vi "Write Options.vi"(8 "error in (no error)":errorcluster, 10 "WebSocket Options":T1, 11 "Websocket Handler in":refnum<class "Websocket Handler.lvclass">) -> (0 "error out":errorcluster, 3 "Websocket Handler out":refnum<class "Websocket Handler.lvclass">)   [LabVIEW 2020, in "wamplv.lvlib" / "Websocket Handler.lvclass"]
uses:
  Websocket Handler.lvclass
  Options.ctl
  Headers.ctl
  Websocket Handler.lvclass/Websocket Handler.ctl
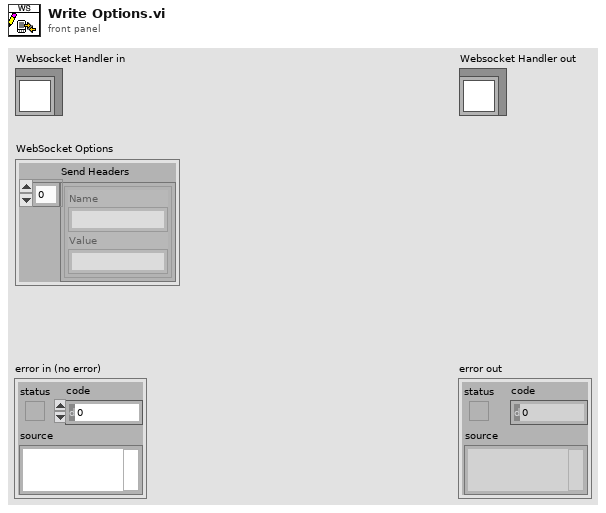
[diagram p1: front panel]
types:
  T1 = typedef "wamplv.lvlib/Websocket Handler.lvclass/Options.ctl" = cluster{"Send Headers":T2[]}
  T2 = typedef "wamplv.lvlib/Websocket Handler.lvclass/Headers.ctl" = cluster{"Name":string, "Value":string}
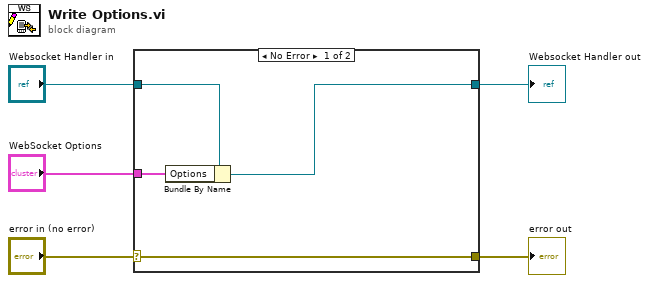
[diagram p0: block diagram]
diagram:
  n1 = case shown="No Error" "error in (no error)" {
    selector: "error in (no error)" -> [w6 w10]
    tunnel: [w6 w10] -> w1
    tunnel: [w7 w11] -> w3
    tunnel: "Websocket Handler in" -> [w9 w11]
    tunnel: "WebSocket Options" -> [w8 _]
    frame No Error {
      n2 = Bundle By Name(cluster=w9, "Options"=w8) -> (w7:refnum<class "Websocket Handler.lvclass">)
    }
    frame Error {
    }
  }
  "error out" <- w1
  "Websocket Handler out" <- w3
